vi "V0.vi"() -> ()   [LabVIEW 2021]
panel:
  in  "GPIB name":string
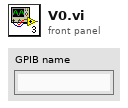
[diagram p1: front panel]
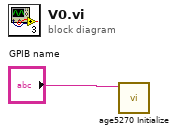
[diagram p0: block diagram]
diagram:
  n1 = call <instrlib>:"age5270 Initialize.vi"("instrdesc"="GPIB name") -> ()  [unwired: 8 in, 3 out]
